vi "Destroy User Event.vi"(8 "error in (no error)":errorcluster, 11 "Camera Controller in":refnum<class "Camera Controller.lvclass">) -> (0 "error out":errorcluster, 3 "Camera Controller out":refnum<class "Camera Controller.lvclass">)   [LabVIEW 2019, in "Camera Controller.lvlib" / "Camera Controller.lvclass"]
uses:
  Camera Controller.lvclass
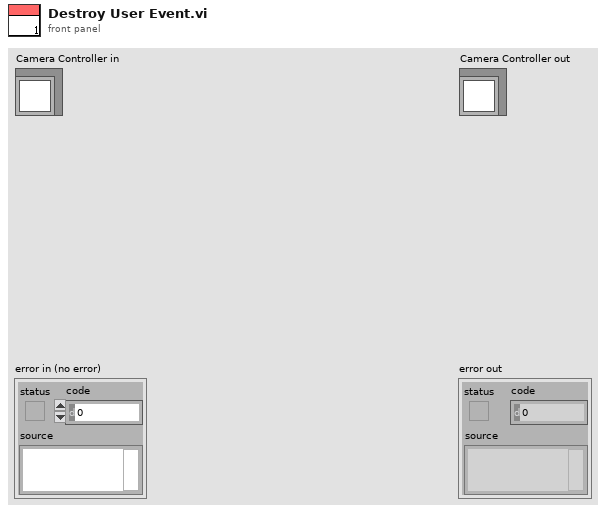
[diagram p1: front panel]
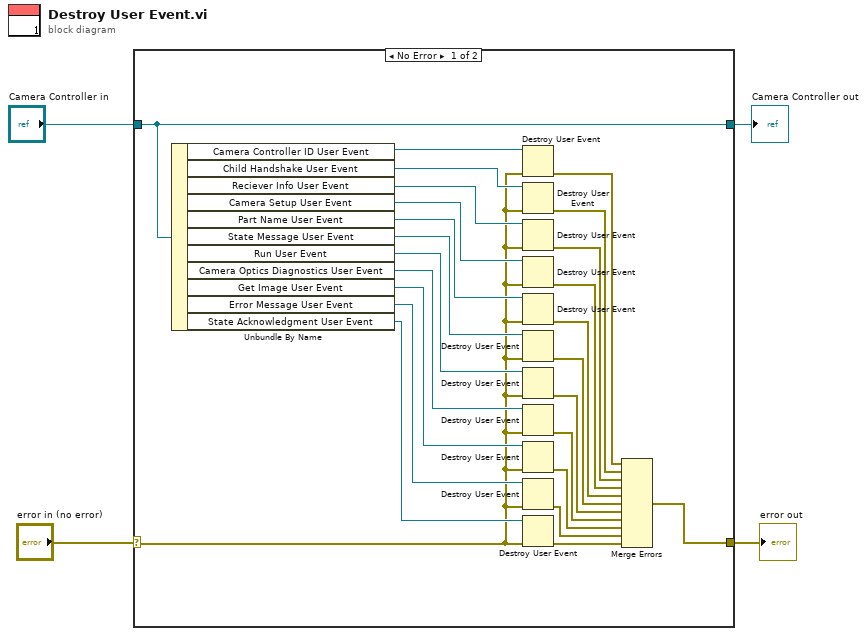
[diagram p0: block diagram]
diagram:
  n1 = case shown="No Error" "error in (no error)" {
    selector: "error in (no error)" -> [w5 w31]
    tunnel: [w6 w31] -> w3
    tunnel: [w18 w30] -> w1
    tunnel: "Camera Controller in" -> [w18 w30]
    frame No Error {
      n2 = Unbundle By Name(w18) -> ("Camera Controller ID User Event"=w17:refnum<user-event>, "Child Handshake User Event"=w16:refnum<user-event>, "Reciever Info User Event"=w7:refnum<user-event>, "Camera Setup User Event"=w8:refnum<user-event>, "Part Name User Event"=w9:refnum<user-event>, "State Message User Event"=w10:refnum<user-event>, "Run User Event"=w11:refnum<user-event>, "Camera Optics Diagnostics User Event"=w12:refnum<user-event>, "Get Image User Event"=w13:refnum<user-event>, "Error Message User Event"=w14:refnum<user-event>, "State Acknowledgment User Event"=w15:refnum<user-event>)
      n3 = Destroy User Event(user event=w17, error in=w5) -> (error out=w19:errorcluster)
      n4 = Destroy User Event(user event=w16, error in=w5) -> (error out=w20:errorcluster)
      n5 = Destroy User Event(user event=w7, error in=w5) -> (error out=w21:errorcluster)
      n6 = Destroy User Event(user event=w8, error in=w5) -> (error out=w22:errorcluster)
      n7 = Destroy User Event(user event=w9, error in=w5) -> (error out=w23:errorcluster)
      n8 = Destroy User Event(user event=w10, error in=w5) -> (error out=w24:errorcluster)
      n9 = Destroy User Event(user event=w11, error in=w5) -> (error out=w25:errorcluster)
      n10 = Destroy User Event(user event=w12, error in=w5) -> (error out=w26:errorcluster)
      n11 = Destroy User Event(user event=w13, error in=w5) -> (error out=w27:errorcluster)
      n12 = Destroy User Event(user event=w14, error in=w5) -> (error out=w28:errorcluster)
      n13 = Destroy User Event(user event=w15, error in=w5) -> (error out=w29:errorcluster)
      n14 = Merge Errors(w19, w20, w21, w22, w23, w24, w25, w26, w27, w28, w29) -> (w6:errorcluster)
    }
    frame Error {
    }
  }
  "error out" <- w3
  "Camera Controller out" <- w1
